vi "Create Folder Shot.vi"(6 "Folders to Exclude":string[](array[string]), 8 "error in (no error)":errorcluster, 10 "Log File Path (*.txt)":path, 11 "Directory Path":path) -> (0 "error out":errorcluster, 3 "Folder Shot":T1[](array[typedef]))   [LabVIEW 2014, in "SLL File IO.lvlib"]
doc: "Create a FolderShot File for the provided Folder Path.\n\nFor each file, it calculates the CRC and stores them in the log file."
uses:
  SLL File IO.lvlib
  _Typedefs/Folder Shot Element.ctl
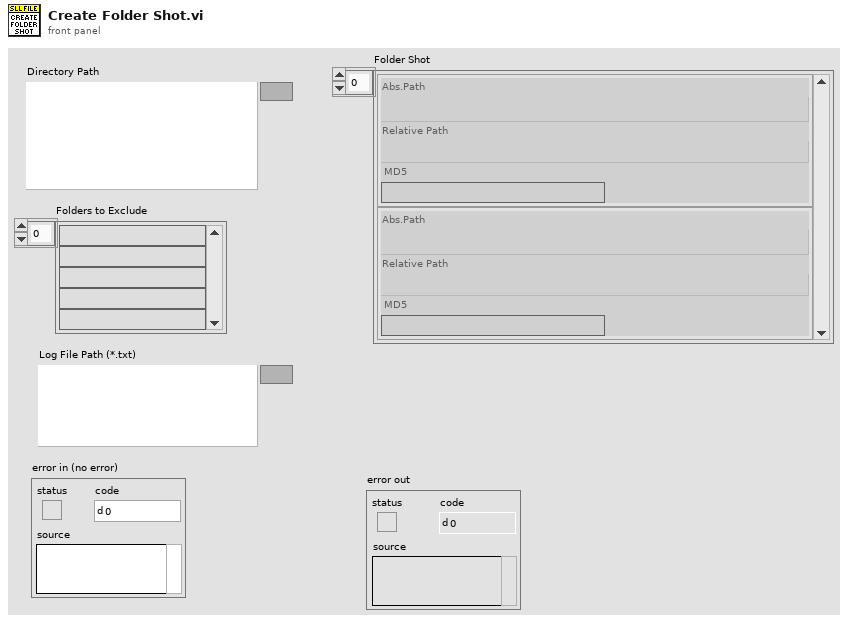
[diagram p1: front panel]
types:
  T1 = typedef "SLL File IO.lvlib/Folder Shot Element.ctl" = cluster{"Abs.Path":path, "Relative Path":path, "MD5":string}
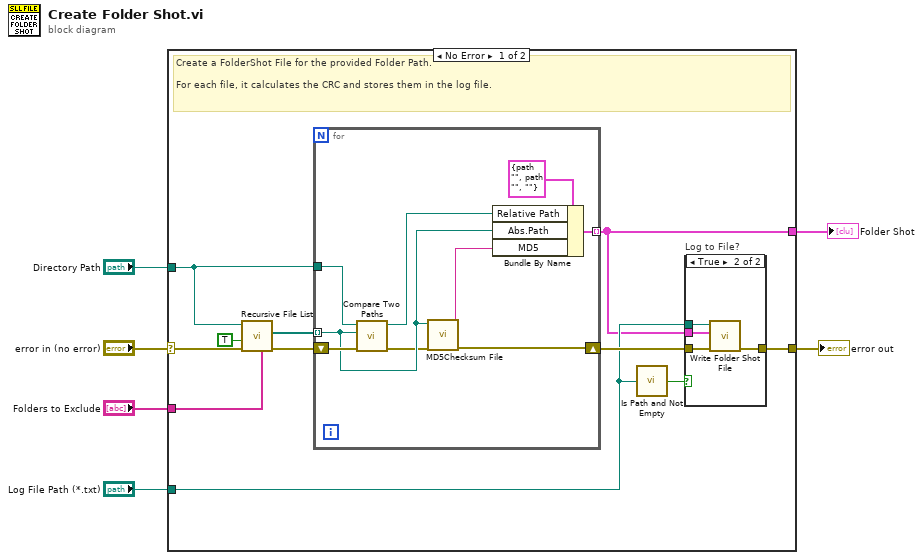
[diagram p0: block diagram]
diagram:
  n1 = case shown="No Error" "error in (no error)" {
    selector: "error in (no error)" -> [w17 w32]
    tunnel: [w10 w32] -> w5
    tunnel: "Directory Path" -> [w12 _]
    tunnel: [w8 _] -> w3
    tunnel: "Folders to Exclude" -> [w11 _]
    tunnel: "Log File Path (*.txt)" -> [w9 _]
    frame No Error {
      # "Create a FolderShot File for the provided Folder Path.\n\nFor each file, it calculates the CRC and stores them in the log file."
      n2 = call <vilib>:"Recursive File List.vi"("Folders to Exclude"=w11, "error in (no error)"=w17, "Continue Recursing on Error? (F)"=TRUE, "Folder Path"=w12) -> ("error out"=w15:errorcluster, "All Files in Dir"=w13:path[])  [unwired: 3 in, 3 out]
      n3 = for {
        shift-right: [w24] -> w14
        shift-left: w15 -> [w28]
        tunnel: w13 -> [w27] mode=indexing
        tunnel: w12 -> [w31]
        tunnel: [w23] -> w8 mode=indexing
        n4 = call <vilib>:"Compare Two Paths.vi"("error in (no error)"=w28, "Path 2"=w27, "Path 1"=w31) -> ("error out"=w25:errorcluster, "Relative Path from 1 to 2"=w29:path)  [unwired: 5 in, 2 out]
        n5 = call <vilib>:"MD5Checksum File.vi"("error in (no error)"=w25, "Path"=w27) -> ("error out"=w24:errorcluster, "MD5 message-digest"=w26:string)  [unwired: 8 in]
        n6 = Bundle By Name(cluster=T1 {"Abs.Path"=path "", "Relative Path"=path "", "MD5"=""} ("Folder Shot Element"), "Relative Path"=w29, "Abs.Path"=w27, "MD5"=w26) -> (w23:T1)
      }
      n7 = call <vilib>:"Is Path and Not Empty.vi"("path"=w9) -> ("Is Path and Not Empty?"=w7:bool)  [unwired: 4 in]
      n8 = case "Log to File?" shown="True" w7 {
        tunnel: w14 -> [w18 w22]
        tunnel: [w18 w21] -> w10
        tunnel: w9 -> [_ w20]
        tunnel: w8 -> [_ w19]
        frame False {
        }
        frame True {
          n9 = call "Write Folder Shot File.vi"("error in (no error)"=w22, "Folder Shot"=w19, "Log Path"=w20) -> ("error out"=w21:errorcluster)  [unwired: 8 in]
        }
      }
    }
    frame Error {
    }
  }
  "error out" <- w5
  "Folder Shot" <- w3
